vi "Save Preferences.vi"(2 "Bookmarks Groupings":T1, 3 "Graveyward Window In":refnum<vi>) -> (1 "Graveyard Window Out":refnum<vi>)   [LabVIEW 2018, in "Bookmark Manager.lvlib"]
uses:
  Bookmark Manager.lvlib
  Controls/Bookmarks Groups.ctl
  Parameter Keys.vi
  <resource>/dialog/lvconfig.llb/LV Config Write String.vi
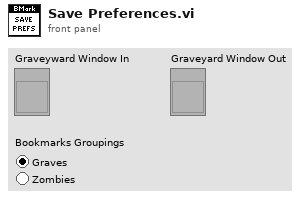
[diagram p1: front panel]
types:
  T1 = typedef "Bookmark Manager.lvlib/Bookmarks Groups.ctl" = enum32{"Graves", "Zombies"}
  T2 = typedef "LVRectTypeDef.ctl" = cluster{"Left":i16, "Top":i16, "Right":i16, "Bottom":i16}
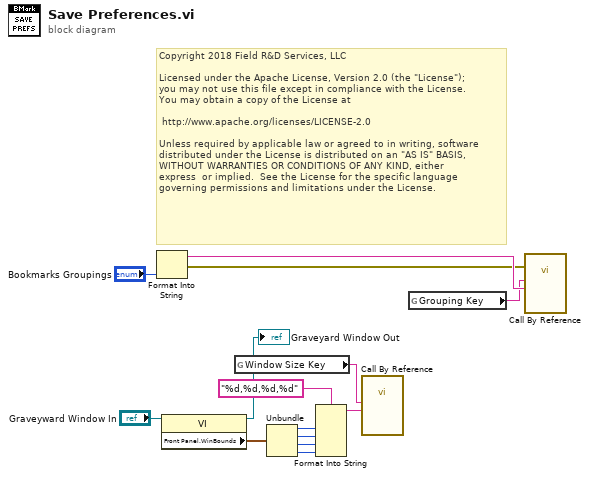
[diagram p0: block diagram]
diagram:
  # "Copyright 2018 Field R&D Services, LLC\n\nLicensed under the Apache License, Version 2.0 (the \"License\");\nyou may not use this file except in compliance with the License.\nYou may obtain a copy of the License at\n\n\thttp://www.apache.org/licenses/LICENSE-2.0\n\nUnless required by applicable law or agreed to in writing, software\ndistributed under the License is distributed on an \"AS IS\" BASIS,\nWITHOUT WARRANTIES OR CONDITIONS OF ANY KIND, either \nexpress  or implied.  See the License for the specific language \ngoverning permissions and limitations under the License."
  n1 = Format Into String("Bookmarks Groupings") -> (resulting string=w5:string, error out=w4:errorcluster)  [unwired: 3 in]
  n2 = property class="VI"(reference="Graveyward Window In") -> (reference out=→"Graveyard Window Out":refnum<vi>, "Front Panel.WinBounds"=w14:T2)  [unwired: 1 in, 1 out]
  n3 = global read "Parameter Keys.vi" "Window Size Key"() -> (w1:string)
  n4 = Unbundle(w14) -> ("Left"=w8:i16, "Top"=w9:i16, "Right"=w10:i16, "Bottom"=w11:i16)
  n5 = Format Into String(format string="%d,%d,%d,%d", w8, w9, w10, w11) -> (resulting string=w13:string)  [unwired: 2 in, 1 out]
  n6 = call-by-ref "?"("value"=w13, "key"=w1) -> ()  [unwired: 3 in, 7 out]
  n7 = global read "Parameter Keys.vi" "Grouping Key"() -> (w2:string)
  n8 = call-by-ref "?"(error in=w4, "value"=w5, "key"=w2) -> ()  [unwired: 2 in, 7 out]
